vi "PhotonCounterV2.vi"() -> ()   [LabVIEW 2012]
doc: "This example demonstrates how to generate and acquire data up to eight channels using an NI 6587 adapter module. It generates either a constant value or a digital count-up pattern on the first eight even, odd, upper, or lower numbered channels of the DDC connector, and then acquires that pattern on the first eight odd, even, lower, or upper (respectively) numbered channels of the DDC connector. The data is generated on one cycle of the single-cycle timed loop and acquired on the next cycle of the loop. To properly verify the waveforms in this example, you must connect the first eight channels to the other eight channels on the DDC connector. For example, if you choose the Even to Odd Channel Configuration, connect the even numbered channels to the odd numbered channels (DIO 0 -> DIO 1, DIO 2 -> DIO 3,...DIO 14 -> DIO 15).\nThis getting started example is intended for lower clock rates depending on your setup. For high speed applications, refer to the Serdes Channel or Serdes Connector examples."
uses:
  <vilib>/Platform/TimedLoop/XDataNode/timing_clust.ctl
  <vilib>/Platform/TimedLoop/XDataNode/nitl_modes.ctl
  <vilib>/Platform/TimedLoop/XDataNode/wakeup.ctl
  <vilib>/rvi/Emulation/niFpgaSctlEmulationRegisterWithScheduler.vi
  <vilib>/rvi/eio/common/nirviEmuTemplateMethod_errors.vi
  <vilib>/rvi/Emulation/niFpgaSctlEmulationScheduler.vi
  <vilib>/rvi/FIFO/Fifo_Resource/nirvififoEmulationSetSize.vi
  <vilib>/rvi/DataTransferAndStorage/Container/Common/niFpgaContainerGetUniqueNameForEmu.vi
  <vilib>/rvi/errors/niFpgaSetErrorForExecOnDevCompSimple.vi
  <vilib>/rvi/eio/common/nirviEmuReportErrorAndStop.vi
  <vilib>/rvi/Emulation/niFpgaSctlEmulationFifoFullMgr.vi
  <vilib>/rvi/Emulation/niFpgaSctlEmulationResourceMgr.vi
  <vilib>/rvi/interface/RandomDataEmulation/nirviRandomDataFPGAFIFO.vi
  <vilib>/rvi/interface/RandomDataEmulation/niFpgaRandomDataHandleErrors.vi
  <vilib>/rvi/Emulation/niFpgaSctlEmulationGlobalWrite.vi
  <vilib>/Platform/TimedLoop/XDataNode/XDataNode.xnode
  <vilib>/eio/EIONode/EIONode.xnode
  <vilib>/rvi/DataTransferAndStorage/Container/XNode/niFpgaContainer.xnode
  <vilib>/rvi/FIFO/Fifo_Resource/nirvififoEmulationClear.vi
  <vilib>/rvi/FIFO/Fifo_Resource/nirvififoEmulationWrite.vi
  <vilib>/rvi/FIFO/Fifo_Resource/nirvififoEmulationRead.vi
  <vilib>/rvi/interface/RandomDataEmulation/nirviRandomDataFpgaReadWriteTemplate.vi
  <vilib>/Platform/TimedLoop/XDataNode/XDNodeRunTimeDep.lvlib
panel:
  in  "Samples per line":u32=16960
  out "ToHost FIFO Overflow Ch2":bool
  in  "Counting mode":bool
  in  "Samples per pixel Acq":u16=16960
  in  "Clear Interloop FIFOs":bool
  in  "Acquire continuously":bool=TRUE
  in  "Requested pixels":u32=1000000
  out "Acquiring":bool
  in  "Wait for trigger":bool
  out "Interloop FIFO overflow":bool
  in  "Samples per pixel":u16=16960
  out "Onboard_Clock_Ready":bool
  in  "Onboard_Clock_Write_Data":u16
  in  "Onboard_Clock_Write":bool
  in  "Clock Source":u8(ring)=3 items=["Tristate"=0, "Sync Clock (PXIe only)"=2, "Adapter Module Onboard Clock"=3, "Strobe from Crosspoint Switch"=4, "Strobe Bypass"=5]
  in  "Xpoint_Switch_Write":bool
  out "Interloop FIFO timeout":bool
  out "ToHost FIFO Overflow Ch1":bool
  in  "Acquire":bool
  in  "Acq_Reset":bool
  out "Xpoint_Switch_Ready":bool
  in  "Commit":bool
  # "6587 IO module configuration"
  # "Acquisition control"
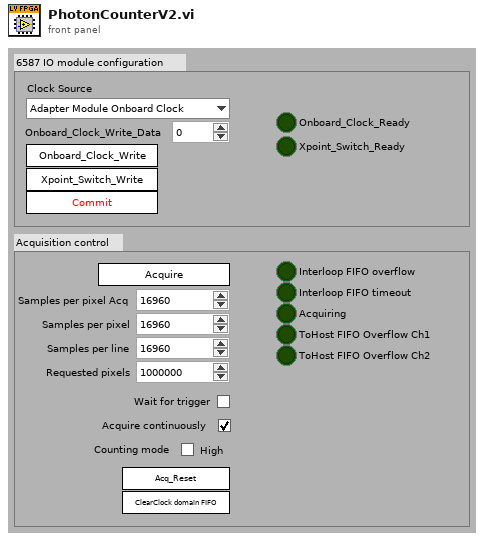
[diagram p1: front panel]
types:
  T1 = typedef "XDNodeRunTimeDep.lvlib/timing_clust.ctl" = cluster{"Expected End [f-1]":u64, "Actual End [f-1]":u64, "Finished Late? [f-1]":bool, "Expected End [i-1]":u64, "Actual End [i-1]":u64, "Finished Late? [i-1]":bool, "Expected Start [i]":u64, "Actual Start [i]":u64, "Expected Start [f]":u64, "Actual Start [f]":u64, "Source Name":string, "Structure Name":string, "Period":i64, "Deadline":i64, "Offset":i64, "Start":i64, "Priority":i32, "Timeout":i32, "Mode":T2, "Wakeup Reason":T3, "Error":errorcluster, "Source Type":string, "Secondary Source Type":string, "Global End Time":u64, "Global Start Time":u64, "Frame Duration":u64, "Iteration Duration":u64, "Assigned CPU":i32, "I/O Scan Engine Mode":u32}
  T2 = typedef "XDNodeRunTimeDep.lvlib/nitl_modes.ctl" = enum32{"No Change", "Process missed periods, maintain original phase", "Discard missed periods, maintain original phase", "Process missed periods, ignore original phase", "Discard missed periods, ignore original phase"}
  T3 = typedef "XDNodeRunTimeDep.lvlib/wakeup.ctl" = enum32{"Normal", "Aborted", "Asynchronous wakeup", "Timing source error", "Timed loop error", "Timeout"}
  T4 = cluster{"IO Module\\LVDS_Ch1_Rd":u16, "IO Module\\LVDS_Ch2_Rd":u16}
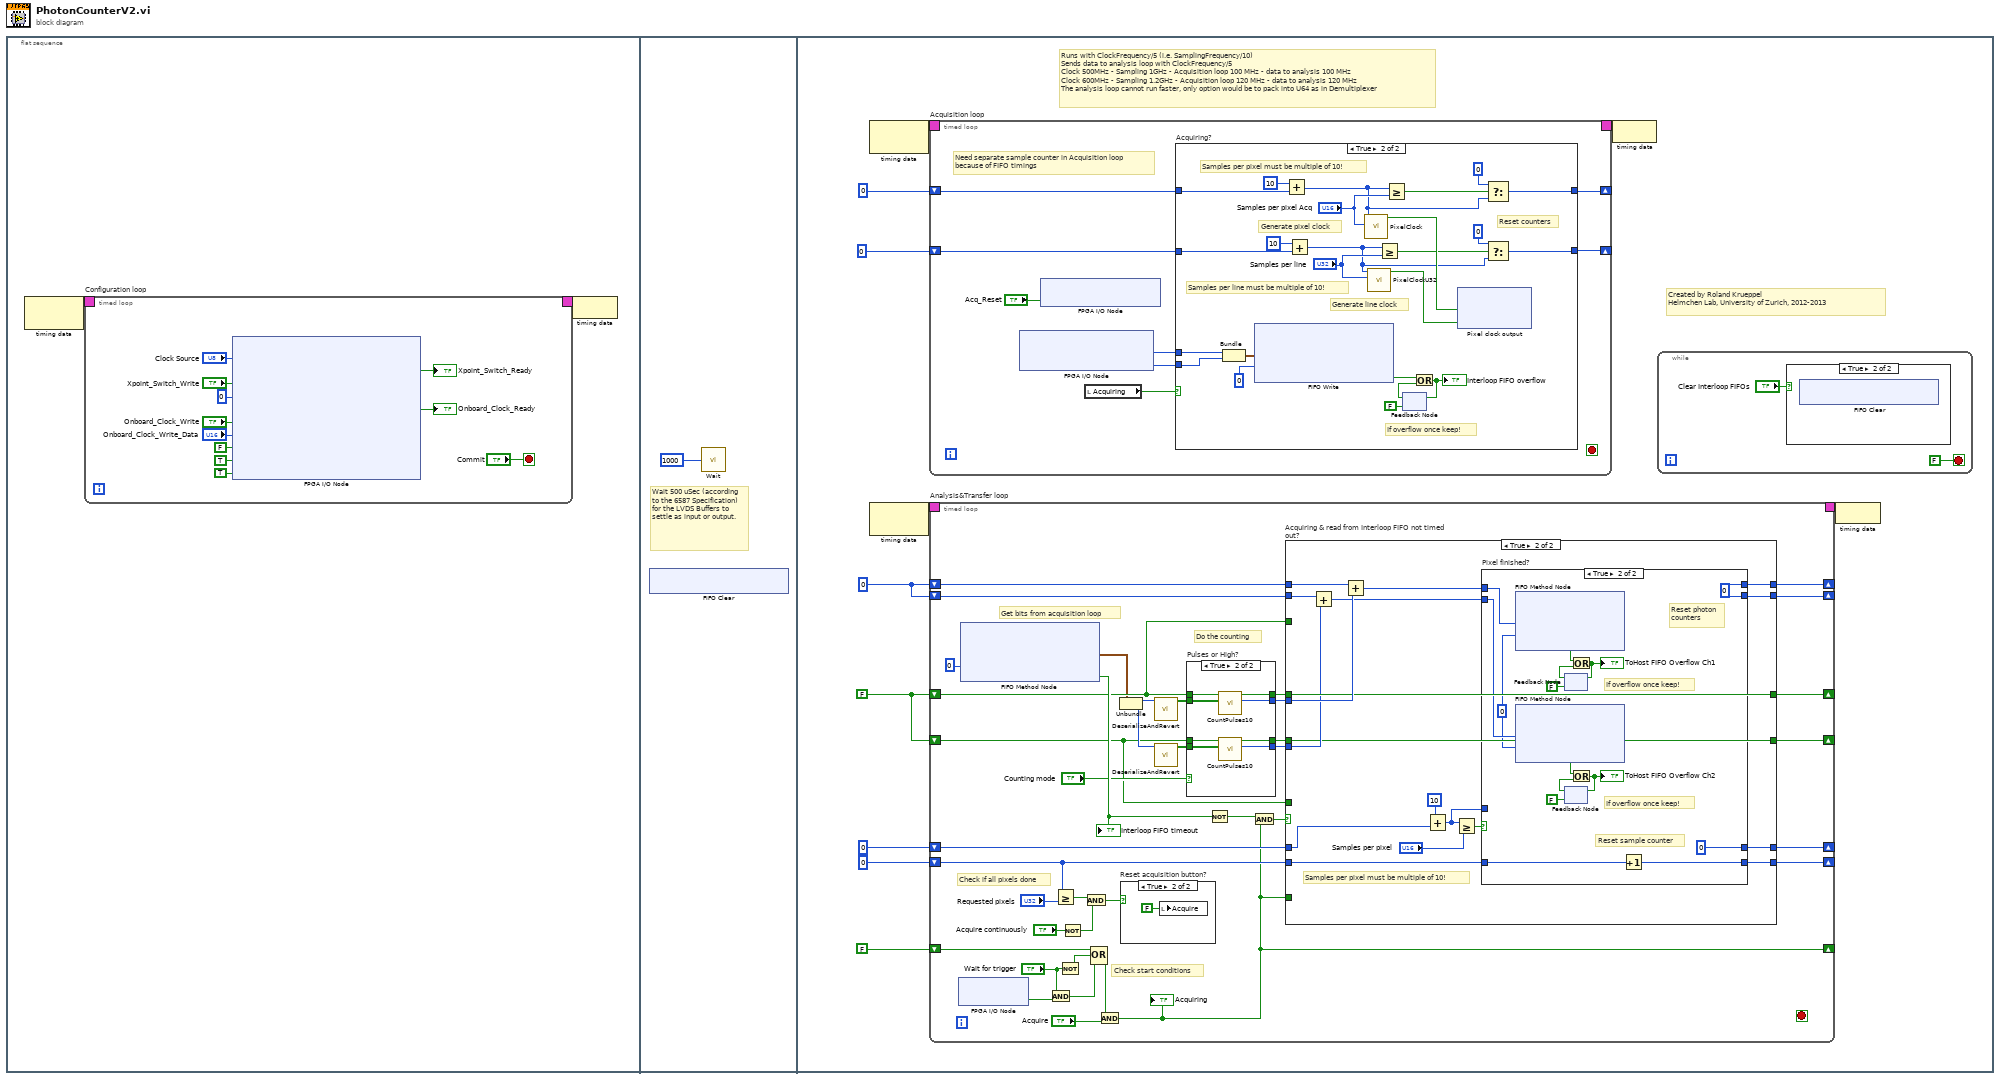
[diagram p0: block diagram]
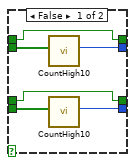
[diagram p3: hidden frame]
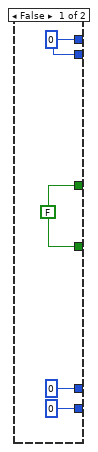
[diagram p6: hidden frame]
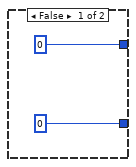
[diagram p8: hidden frame]
diagram:
  n1 = flat-sequence {
    frame #0 {
      n2 = node-c288() -> (w2:T1)  [unwired: 1 in]
      n3 = timed-loop "Configuration loop" {
        timing: w2 -> [_]
        timing-out: [_] -> w1
        stop <- "Commit" stop-if-true
        n4 = xnode "FPGA I/O Node"("IO Module\\Acq_IO_Clock_Source"="Clock Source", "IO Module\\Xpoint_Switch_Write"="Xpoint_Switch_Write", "IO Module\\LVDS_Data_Dir"=u16 0 ("IO Module\\LVDS_Data_Dir"), "IO Module\\Onboard_Clock_Write"="Onboard_Clock_Write", "IO Module\\Onboard_Clock_Write_Data"="Onboard_Clock_Write_Data", "IO Module\\SE_PFI0_WE"=FALSE ("IO Module\\SE_PFI0_WE"), "IO Module\\SE_PFI1_WE"=TRUE ("IO Module\\SE_PFI1_WE"), "IO Module\\LVDS_ClockOut_Enable"=TRUE ("IO Module\\LVDS_ClockOut_Enable")) -> ("IO Module\\Xpoint_Switch_Ready"=→"Xpoint_Switch_Ready":bool, "IO Module\\Onboard_Clock_Ready"=→"Onboard_Clock_Ready":bool)  [unwired: 10 in, 10 out]
      }
      n5 = node-c288(w1) -> ()
    }
    frame #1 {
      # "Wait 500 uSec (according to the 6587 Specification) for the LVDS Buffers to settle as input or output."
      n6 = xnode ("FIFO Clear")() -> ()  [unwired: 1 in, 1 out]
      n7 = call "Wait"("Count(uSec)"=u32 1000 ("Wait (uSec)")) -> ()  [unwired: 1 out]
    }
    frame #2 {
      w20 = FALSE ("New last sample")
      w21 = u16 0
      # "Runs with ClockFrequency/5 (i.e. SamplingFrequency/10)\nSends data to analysis loop with ClockFrequency/5\nClock 500MHz - Sampling 1GHz - Acquisition loop 100 MHz - data to analysis 100 MHz\nClock 600MHz - Sampling 1.2GHz - Acquisition loop 120 MHz - data to analysis 120 MHz\nThe analysis loop cannot run faster, only option would be to pack into U64 as in Demultiplexer"
      # "Created by Roland Krueppel\nHelmchen Lab, University of Zurich, 2012-2013"
      n8 = node-c288() -> (w29:T1)  [unwired: 1 in]
      n9 = node-c288() -> (w27:T1)  [unwired: 1 in]
      n10 = timed-loop "Acquisition loop" {
        timing: w29 -> [_]
        timing-out: [_] -> w28
        shift-right: [w152] -> _
        shift-left: u16 0 ("t") -> [w153]
        shift-right: [w150] -> _
        shift-left: u32 0 -> [w151]
        stop <- _ stop-if-true
        # "Need separate sample counter in Acquisition loop\nbecause of FIFO timings"
        n11 = xnode "FPGA I/O Node"() -> ("IO Module\\LVDS_Ch1_Rd"=w156:u16, "IO Module\\LVDS_Ch2_Rd"=w154:u16)  [unwired: 2 in, 2 out]
        n12 = xnode "FPGA I/O Node"("IO Module\\Acq_Reset"="Acq_Reset") -> ()  [unwired: 1 in, 1 out]
        n13 = local read "Acquiring"() -> (w155:bool)
        n14 = case "Acquiring?" shown="True" w155 {
          tunnel: w156 -> [_ w175]
          tunnel: w154 -> [_ w174]
          tunnel: w153 -> [_ w180]
          tunnel: [u16 0 ("t") w179] -> w152
          tunnel: w151 -> [_ w167]
          tunnel: [u32 0 ("t") w163] -> w150
          frame False {
          }
          frame True {
            # "Samples per line must be multiple of 10!"
            # "Generate line clock"
            # "If overflow once keep!"
            # "Reset counters"
            # "Generate pixel clock"
            # "Samples per pixel must be multiple of 10!"
            n15 = Bundle("IO Module\\LVDS_Ch1_Rd"=w175, "IO Module\\LVDS_Ch2_Rd"=w174) -> (w173:T4)  [unwired: 1 in]
            n16 = xnode ("FIFO Write")("Element"=w173, "Timeout"=0) -> ("Timed Out?"=w171:bool)  [unwired: 1 in, 1 out]
            n17 = Add(x=u16 10 ("y"), y=w180) -> (x+y=w177:u16)
            n18 = Add(x=u32 10, y=w167) -> (x+y=w162:u32)
            n19 = call "PixelClock.vi"("Samples per pixel"="Samples per pixel Acq", "Sample counter"=w177) -> ("Pixel clock"=w181:bool)  [unwired: 9 in]
            n20 = call "PixelClockU32.vi"("Samples per pixel"="Samples per line", "Sample counter"=w162) -> ("Pixel clock"=w160:bool)  [unwired: 9 in]
            n21 = Greater Or Equal?(x=w162, y="Samples per line") -> (x >= y?=w164:bool)
            n22 = Greater Or Equal?(x=w177, y="Samples per pixel Acq") -> (x >= y?=w176:bool)
            n23 = feedback #1(FALSE) -> (w168:bool)
            n24 = Or(x=w171, y=w168) -> (x .or. y?=w170:bool)
            "Interloop FIFO overflow" <- w170
            n25 = feedback-in #1(w170) -> ()
            n26 = xnode "Pixel clock output"("Pixel clock"=w181, "Line clock"=w160) -> ()  [unwired: 2 in, 2 out]
            n27 = Select(t=u16 0, s=w176, f=w177) -> (s? t:f=w179:u16)
            n28 = Select(t=u32 0, s=w164, f=w162) -> (s? t:f=w163:u32)
          }
        }
      }
      n29 = timed-loop "Analysis&Transfer loop" {
        timing: w27 -> [_]
        timing-out: [_] -> w26
        shift-right: [w62] -> _
        shift-left: w21 -> [w70]
        shift-right: [w69] -> _
        shift-left: u16 0 -> [w68]
        shift-right: [w67] -> _
        shift-left: u32 0 -> [w63]
        shift-right: [w48] -> _
        shift-left: FALSE ("New last sample") -> [w65]
        shift-right: [w44] -> _
        shift-left: w20 -> [w43]
        shift-right: [w34] -> _
        shift-left: w21 -> [w41]
        shift-right: [w32] -> _
        shift-left: w20 -> [w33]
        stop <- _ stop-if-true
        # "Do the counting"
        # "Get bits from acquisition loop"
        # "Check start conditions"
        # "Check if all pixels done"
        n30 = xnode "FPGA I/O Node"() -> ("TriggerIn"=w53:bool)  [unwired: 1 in, 1 out]
        n31 = xnode ("FIFO Method Node")("Timeout"=0) -> ("Element"=w40:cluster{"Ch0":u16, "Ch1":u16}, "Timed Out?"=w49:bool)  [unwired: 1 in, 1 out]
        "Interloop FIFO timeout" <- w49
        n32 = And(x="Wait for trigger", y=w53) -> (x .and. y?=w52:bool)
        n33 = Greater Or Equal?(x=w63, y="Requested pixels") -> (x >= y?=w60:bool)
        n34 = Not(x="Wait for trigger") -> (.not. x?=w66:bool)
        n35 = Not(x="Acquire continuously") -> (.not. x?=w58:bool)
        n36 = And(x=w60, y=w58) -> (x .and. y?=w61:bool)
        n37 = Compound Arithmetic op=OR(w65, w66, w52) -> (w51:bool)
        n38 = And(x=w51, y="Acquire") -> (x .and. y?=w48:bool)
        "Acquiring" <- w48
        n39 = Unbundle(w40) -> ("Ch0"=w39:u16, "Ch1"=w38:u16)
        n40 = case "Reset acquisition button?" shown="True" w61 {
          frame False {
          }
          frame True {
            n41 = local write "Acquire"(FALSE ("Acquire")) -> ()
          }
        }
        n42 = call "DeserializeAndRevert.vi"("U16 input"=w39) -> ("10bit output"=w47:bool[])  [unwired: 10 in]
        n43 = call "DeserializeAndRevert.vi"("U16 input"=w38) -> ("10bit output"=w37:bool[])  [unwired: 10 in]
        n44 = case "Pulses or High?" shown="True" "Counting mode" {
          tunnel: w47 -> [w76 w84]
          tunnel: [w75 w83] -> w46
          tunnel: [w74 w82] -> w45
          tunnel: w43 -> [w74 w81]
          tunnel: w37 -> [w73 w80]
          tunnel: [w72 w78] -> w35
          tunnel: [w71 w79] -> w36
          tunnel: w33 -> [w71 w77]
          frame False {
            n45 = call "CountHigh10.vi"("10bit input"=w76) -> ("No. of detected high"=w75:u16)  [unwired: 10 in]
            n46 = call "CountHigh10.vi"("10bit input"=w73) -> ("No. of detected high"=w72:u16)  [unwired: 10 in]
          }
          frame True {
            n47 = call "CountPulses10.vi"("10bit input"=w84, "Last sample"=w81) -> ("No. of detected pulses"=w83:u16, "New last sample"=w82:bool)  [unwired: 8 in]
            n48 = call "CountPulses10.vi"("10bit input"=w80, "Last sample"=w77) -> ("No. of detected pulses"=w78:u16, "New last sample"=w79:bool)  [unwired: 8 in]
          }
        }
        n49 = Not(x=w49) -> (.not. x?=w57:bool)
        n50 = And(x=w57, y=w48) -> (x .and. y?=w56:bool)
        n51 = case "Acquiring & read from Interloop FIFO not timed out?" shown="True" w56 {
          tunnel: w70 -> [w98 w126]
          tunnel: [w94 w122] -> w69
          tunnel: w68 -> [w97 w117]
          tunnel: w63 -> [w96 w121]
          tunnel: [w93 w120] -> w67
          tunnel: [w95 w119] -> w62
          tunnel: w46 -> [_ w115]
          tunnel: w48 -> [w92 _]
          tunnel: w45 -> [_ w114]
          tunnel: [w90 w114] -> w44
          tunnel: w43 -> [w91 _]
          tunnel: w41 -> [w87 w113]
          tunnel: w36 -> [_ w109]
          tunnel: w35 -> [_ w112]
          tunnel: [w86 w110] -> w34
          tunnel: w33 -> [w89 _]
          tunnel: [w88 w109] -> w32
          frame False {
            n52 = case "Acquiring?" shown="True" w92 {
              tunnel: w98 -> [_ w108]
              tunnel: w97 -> [_ w107]
              tunnel: w96 -> [_ w106]
              tunnel: [w99 w108] -> w95
              tunnel: [u16 0 w107] -> w94
              tunnel: [u32 0 w106] -> w93
              tunnel: w91 -> [_ w105]
              tunnel: [w100 w105] -> w90
              tunnel: w89 -> [_ w104]
              tunnel: [w100 w104] -> w88
              tunnel: w87 -> [_ w103]
              tunnel: [w99 w103] -> w86
              frame False {
                w100 = FALSE ("New last sample")
                w99 = u16 0
              }
              frame True {
              }
            }
          }
          frame True {
            # "Samples per pixel must be multiple of 10!"
            n53 = Add(x=w113, y=w112) -> (x+y=w111:u16)
            n54 = Add(x=w126, y=w115) -> (x+y=w118:u16)
            n55 = Add(x=u16 10 ("y"), y=w117) -> (x+y=w123:u16)
            n56 = Greater Or Equal?(x=w123, y="Samples per pixel") -> (x >= y?=w124:bool)
            n57 = case "Pixel finished?" shown="True" w124 {
              tunnel: w123 -> [w130 _]
              tunnel: [w130 u16 0] -> w122
              tunnel: w121 -> [w129 w145]
              tunnel: [w129 w144] -> w120
              tunnel: [w128 w139] -> w119
              tunnel: w118 -> [w128 w142]
              tunnel: w111 -> [w127 w141]
              tunnel: [w127 w139] -> w110
              frame False {
              }
              frame True {
                w139 = u16 0
                w140 = 0 ("Timeout")
                # "If overflow once keep!"
                # "If overflow once keep!"
                # "Reset photon\ncounters"
                # "Reset sample counter"
                n58 = xnode ("FIFO Method Node")("Element"=w142, "Timeout"=w140) -> ("Timed Out?"=w138:bool)  [unwired: 1 in, 1 out]
                n59 = xnode ("FIFO Method Node")("Element"=w141, "Timeout"=w140) -> ("Timed Out?"=w132:bool)  [unwired: 1 in, 1 out]
                n60 = feedback #2(FALSE) -> (w136:bool)
                n61 = feedback #3(FALSE) -> (w134:bool)
                n62 = Or(x=w138, y=w136) -> (x .or. y?=w137:bool)
                "ToHost FIFO Overflow Ch1" <- w137
                n63 = feedback-in #2(w137) -> ()
                n64 = Or(x=w132, y=w134) -> (x .or. y?=w131:bool)
                "ToHost FIFO Overflow Ch2" <- w131
                n65 = feedback-in #3(w131) -> ()
                n66 = Increment(x=w145) -> (x+1=w144:u32)
              }
            }
          }
        }
      }
      n67 = node-c288(w28) -> ()
      n68 = while {
        stop <- FALSE stop-if-true
        n69 = case shown="True" "Clear Interloop FIFOs" {
          frame False {
          }
          frame True {
            n70 = xnode ("FIFO Clear")() -> ()  [unwired: 1 in, 1 out]
          }
        }
      }
      n71 = node-c288(w26) -> ()
    }
  }
